vi "Radau5_Norm with Index.vi"(9 "Index of Y":i8[](array[numeric]), 10 "ErrorTolerance":dbl[](array[numeric]), 11 "Local error":dbl[](array[numeric])) -> (3 "Error":dbl)   [LabVIEW 2017, in "NI_DAE.lvlib"]
uses:
  <vilib>/gmath/NI_DAE.lvlib
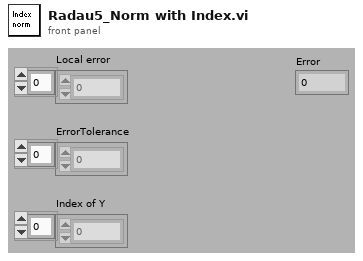
[diagram p1: front panel]
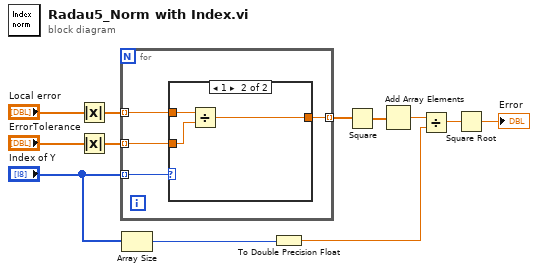
[diagram p0: block diagram]
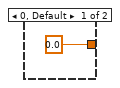
[diagram p2: hidden frame]
diagram:
  n1 = Absolute Value(x="Local error") -> (abs(x)=w11:dbl[])
  n2 = Absolute Value(x="ErrorTolerance") -> (abs(x)=w9:dbl[])
  n3 = for {
    tunnel: "Index of Y" -> [w16] mode=indexing
    tunnel: w11 -> [w15] mode=indexing
    tunnel: w9 -> [w14] mode=indexing
    tunnel: [w13] -> w8 mode=indexing
    n4 = case shown="1" w16 {
      tunnel: w15 -> [_ w20]
      tunnel: w14 -> [_ w19]
      tunnel: [0.0 w18] -> w13
      frame 0, Default {
      }
      frame 1 {
        n5 = Divide(x=w20, y=w19) -> (x/y=w18:dbl)
      }
    }
  }
  n6 = Array Size(array="Index of Y") -> (size(s)=w4:i32)
  n7 = To Double Precision Float(number=w4) -> (double precision float=w3:dbl)
  n8 = Square(x=w8) -> (x^2=w7:dbl[])
  n9 = Add Array Elements(numeric array=w7) -> (sum=w5:dbl)
  n10 = Divide(x=w5, y=w3) -> (x/y=w2:dbl)
  n11 = Square Root(x=w2) -> (sqrt(x)=→"Error":dbl)
